vi "Puff_using_Arduino.vi"() -> (5 "Plug in titles":string[](array[string]), 7 "Plug in values":string[](array[string]))   [LabVIEW 2012]
uses:
  Controls/Post_Process.ctl
  Controls/Setup.ctl
  Globals/Meas_global.vi
panel:
  out "Puff Time used":dbl=1.0 format="%.2g"
  out "EnFlo_Tunnel Metadata:Puff_duration:Sec":dbl=1.0 format="%.2g"
  out "Case Currently On":string="Loop"
  # "Change this value via the ADAM Scan Table"
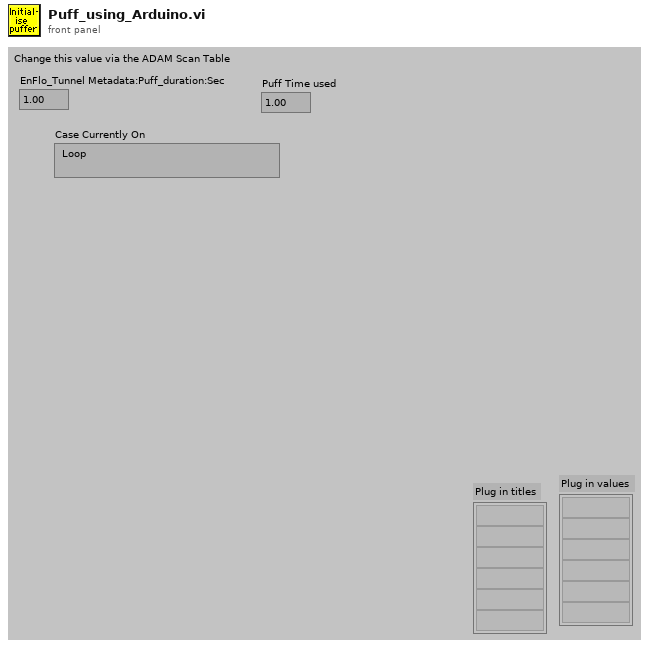
[diagram p1: front panel]
types:
  T1 = typedef "Setup.ctl" = enum16{"Run Program", "Show Setup", "Save Current Setup", "Setup Front Panel"}
  T2 = typedef "Post_Process.ctl" = enum16{"Take New Data", "Post Process Raw Data File"}
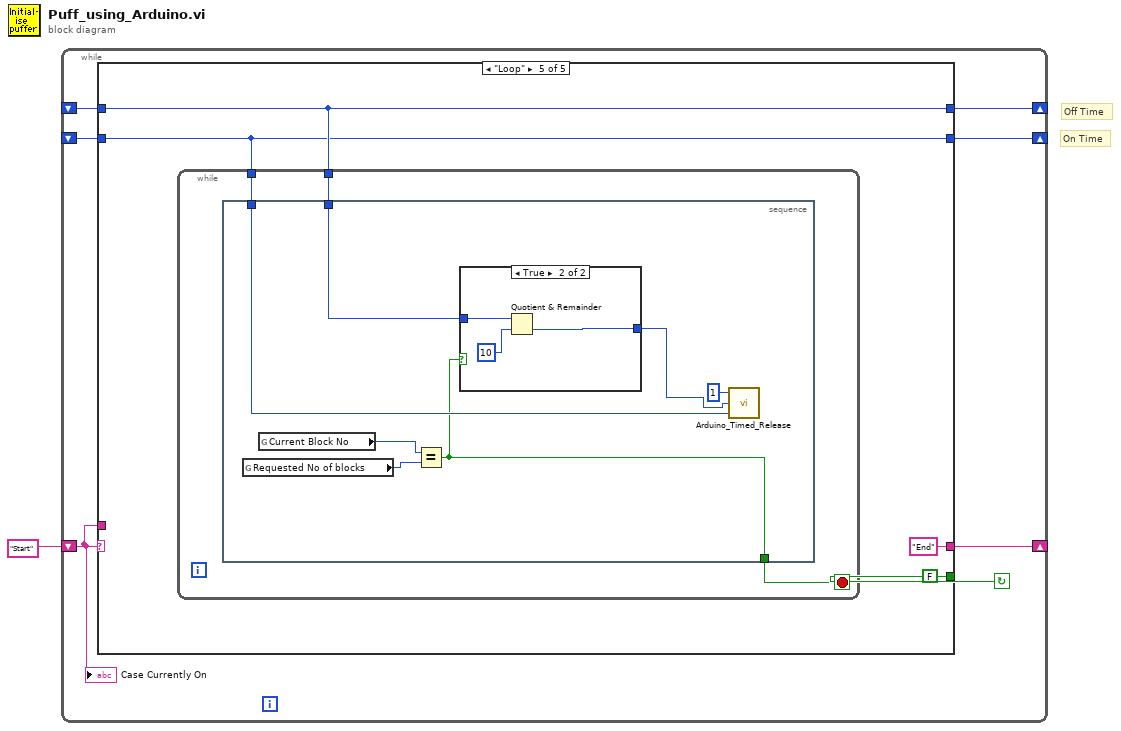
[diagram p0: block diagram]
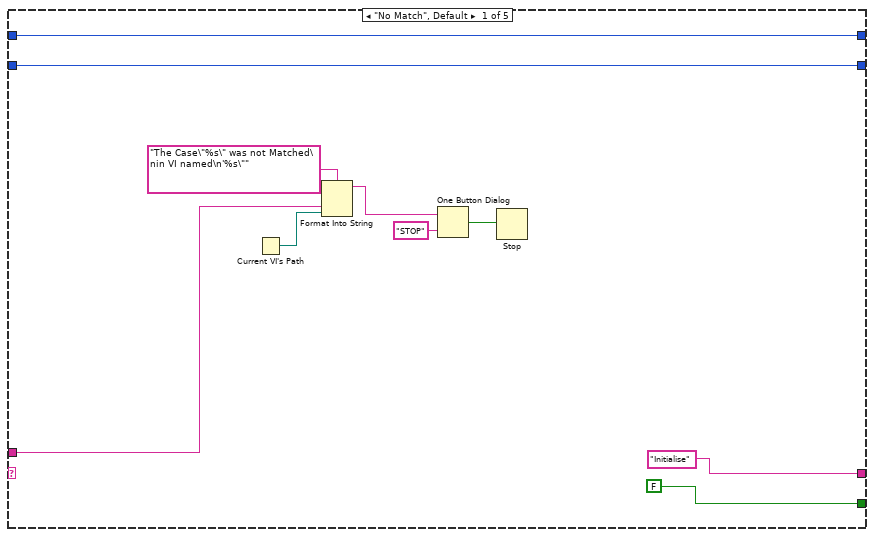
[diagram p2: hidden frame]
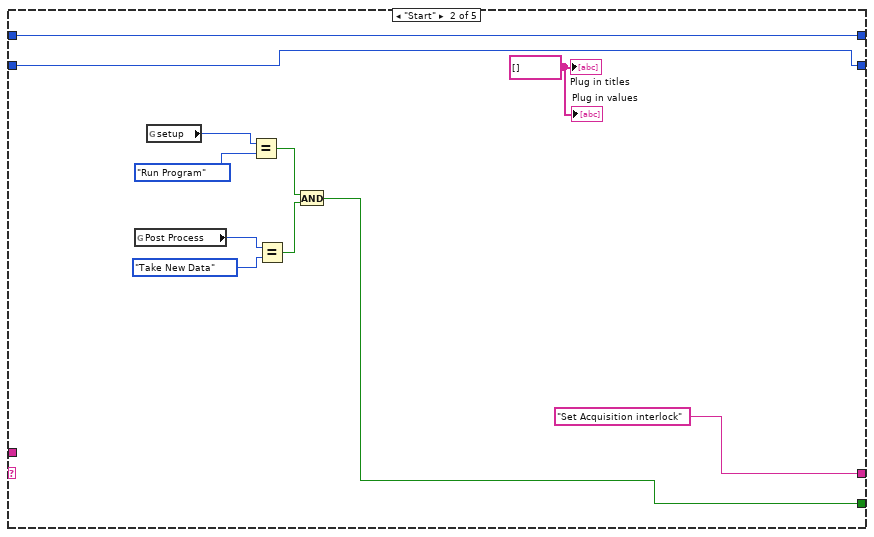
[diagram p3: hidden frame]
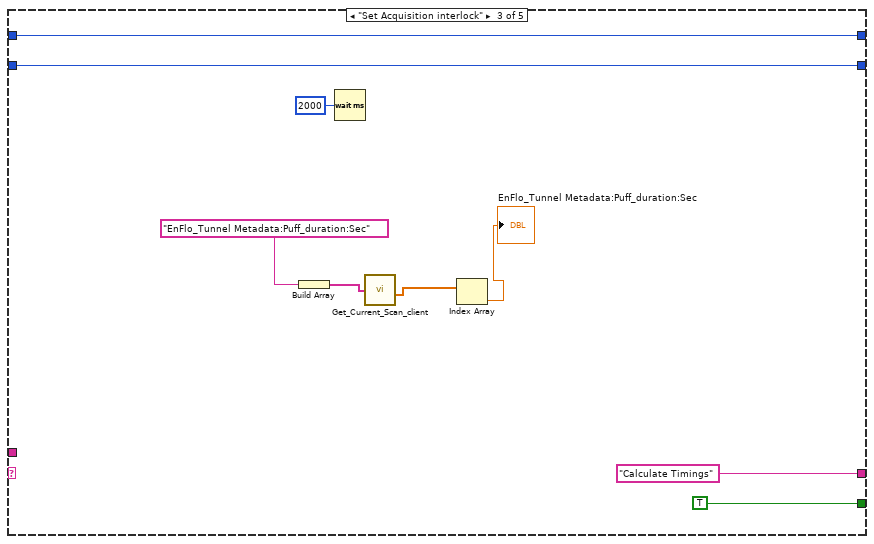
[diagram p4: hidden frame]
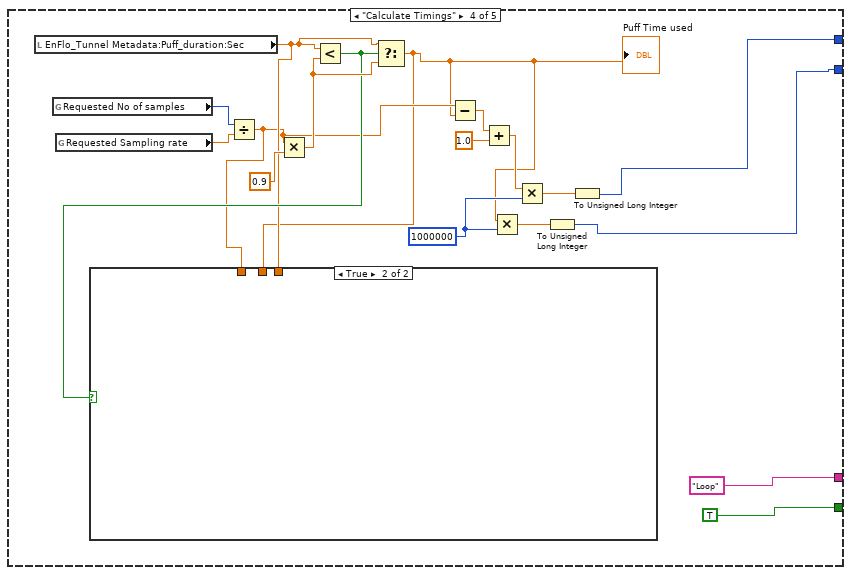
[diagram p5: hidden frame]
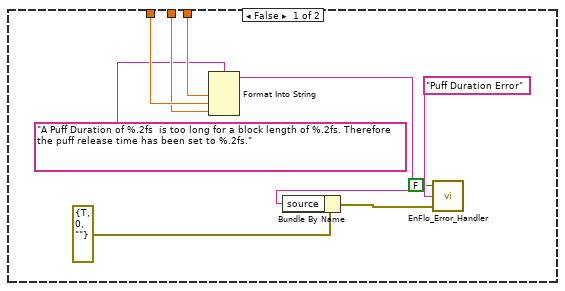
[diagram p6: hidden frame]
diagram:
  # "On Time"
  # "Off Time"
  n1 = while {
    shift-left: "Start" -> [w6]
    shift-right: [w7] -> _
    shift-right: [w5] -> _
    shift-left: _ -> [w4]
    shift-right: [w3] -> _
    shift-left: _ -> [w2]
    stop <- w8 continue-if-true
    n2 = case shown="\"Loop\"" w6 {
      tunnel: [FALSE w21 TRUE ("Command Found") TRUE ("Command Found") FALSE ("Command Found")] -> w8
      tunnel: ["Initialise" "Set Acquisition interlock" "Calculate Timings" "Loop" "End"] -> w7
      tunnel: w6 -> [w13 _ _ _ _]
      tunnel: [w10 w20 w31 w40 w69] -> w5
      tunnel: w4 -> [w10 w20 w31 _ w69]
      tunnel: [w9 w19 w30 w39 w68] -> w3
      tunnel: w2 -> [w9 w19 w30 _ w68]
      frame "No Match", Default {
        n3 = Current VI's Path() -> (path=w12:path)
        n4 = Format Into String(format string="The Case\"%s\" was not Matched\nin VI named\n'%s\"" ("Format String"), w13, w12) -> (resulting string=w16:string)  [unwired: 2 in, 1 out]
        n5 = One Button Dialog(message=w16, button name ("OK")="STOP") -> (true=w14:bool)
        n6 = Stop(stop? (T)=w14) -> ()
      }
      frame "Start" {
        w28 = string[] [] ("Plug in titles")
        n7 = global read "Meas_global.vi" "Post Process"() -> (w23:T2)
        n8 = global read "Meas_global.vi" "setup"() -> (w22:T1)
        n9 = Equal?(x=w22, y=Setup."Run Program") -> (x = y?=w27:bool)
        n10 = Equal?(x=w23, y=Post_Process."Take New Data" ("Post Process")) -> (x = y?=w26:bool)
        n11 = And(x=w27, y=w26) -> (x .and. y?=w21:bool)
        "Plug in values" <- w28
        "Plug in titles" <- w28
      }
      frame "Set Acquisition interlock" {
        n12 = Build Array("EnFlo_Tunnel Metadata:Puff_duration:Sec") -> (w34:string[])
        n13 = Wait (ms)(milliseconds to wait=u32 2000) -> ()  [unwired: 1 out]
        n14 = call "Get_Current_Scan_client.vi"("ADAM Ch Names"=w34) -> ("Numerical Values"=w33:dbl[])  [unwired: 1 in, 2 out]
        n15 = Index Array(array=w33) -> (element=→"EnFlo_Tunnel Metadata:Puff_duration:Sec":dbl)  [unwired: 1 in]
      }
      frame "Calculate Timings" {
        w49 = u32 1000000 ("y")
        n16 = local read "EnFlo_Tunnel Metadata:Puff_duration:Sec"() -> (w44:dbl)
        n17 = global read "Meas_global.vi" "Requested No of samples"() -> (w54:i32)
        n18 = global read "Meas_global.vi" "Requested Sampling rate"() -> (w43:dbl)
        n19 = Divide(x=w54, y=w43) -> (x/y=w42:dbl)
        n20 = Multiply(x=w42, y=0.9) -> (x*y=w52:dbl)
        n21 = Less?(x=w44, y=w52) -> (x < y?=w45:bool)
        n22 = Select(t=w44, s=w45, f=w52) -> (s? t:f=w41:dbl)
        "Puff Time used" <- w41
        n23 = case shown="True" w45 {
          tunnel: w44 -> [w63 _]
          tunnel: w42 -> [w62 _]
          tunnel: w41 -> [w61 _]
          frame False {
            n24 = Format Into String(format string="A Puff Duration of %.2fs  is too long for a block length of %.2fs. Therefore the puff release time has been set to %.2fs.", w63, w62, w61) -> (resulting string=w59:string)  [unwired: 2 in, 1 out]
            n25 = Bundle By Name(cluster=errorcluster {"status"=TRUE, "code"=0, "source"=""} ("error in (no error)"), "source"=w59) -> (w64:errorcluster)
            n26 = call "EnFlo_Error_Handler.vi"("error in (no error)"=w64, "Error Type"="Puff Duration Error", "Dialog Box (T)"=FALSE) -> ()  [unwired: 3 out]
          }
          frame True {
          }
        }
        n27 = Subtract(x=w42, y=w41) -> (x-y=w48:dbl)
        n28 = Add(x=w48, y=1.0) -> (x+y=w46:dbl)
        n29 = Multiply(x=w41, y=w49) -> (x*y=w51:dbl)
        n30 = Multiply(x=w46, y=w49) -> (x*y=w50:dbl)
        n31 = To Unsigned Long Integer(number=w51) -> (unsigned 32bit integer=w39:u32)
        n32 = To Unsigned Long Integer(number=w50) -> (unsigned 32bit integer=w40:u32)
      }
      frame "Loop" {
        n33 = while {
          tunnel: w69 -> [w70]
          tunnel: w68 -> [w72]
          stop <- w71 stop-if-true
          n34 = stacked-sequence {
            tunnel: w72 -> [w78]
            tunnel: [w73] -> w71
            tunnel: w70 -> [w77]
            frame #0 {
              n35 = global read "Meas_global.vi" "Requested No of blocks"() -> (w75:i32)
              n36 = global read "Meas_global.vi" "Current Block No"() -> (w74:i32)
              n37 = Equal?(x=w74, y=w75) -> (x = y?=w73:bool)
              n38 = case shown="True" w73 {
                tunnel: w77 -> [w80 w83]
                tunnel: [w80 w81] -> w76
                frame False {
                }
                frame True {
                  n39 = Quotient & Remainder(x=w83, y=u32 10) -> (floor(x/y)=w81:u32)  [unwired: 1 out]
                }
              }
              n40 = call "Arduino_Timed_Release.vi"("Time to hold source ON (microseconds)"=w78, "Time to hold source OFF (microseconds)"=w76, "Number of cycles"=u16 1) -> ()  [unwired: 2 out]
            }
          }
        }
      }
    }
    "Case Currently On" <- w6
  }
